vi "sub_lidar-range_line.vi"() -> (3 "guide line":cluster{cluster{"x":dbl, "y":dbl}[]})   [LabVIEW 2019]
uses:
  Ctrl/obstacle_info.ctl
panel:
  in  "input cluster":cluster{"h-L":i16, "h-R":i16}
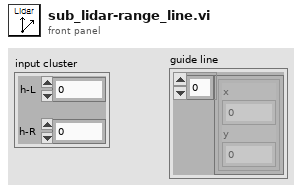
[diagram p1: front panel]
types:
  T1 = typedef "obstacle_info.ctl" = enum16{"init", "read", "obstacle status in", "write limit", "inrange pt-n"}
  T2 = cluster{"h range":cluster{i16, i16}, "v range":cluster{i8, i8}}
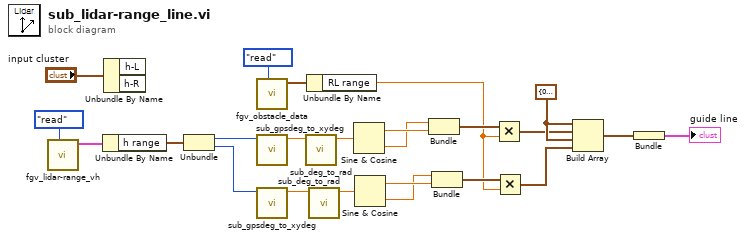
[diagram p0: block diagram]
diagram:
  w22 = cluster{"x":dbl, "y":dbl} {"x"=0.0, "y"=0.0} ("output cluster")
  n1 = call "fgv_lidar-range_vh.vi"("cmd"=enum16{"read", "write"}."read") -> ("VLP16 cfg out"=w4:T2)  [unwired: 10 in]
  n2 = Unbundle By Name(w4) -> ("h range"=w3:cluster{i16, i16})
  n3 = Unbundle By Name("input cluster") -> ()  [unwired: 2 out]
  n4 = Unbundle(w3) -> (w2:i16, w1:i16)
  n5 = call "fgv_obstacle_data.vi"("cmd"=obstacle_info."read") -> ("limit out"=w15:cluster{"RL range":dbl, "Point limit":u16})  [unwired: 7 in, 3 out]
  n6 = call "sub_gpsdeg_to_xydeg.vi"("Heading"=w2) -> ("deg"=w24:dbl)  [unwired: 10 in]
  n7 = call "sub_gpsdeg_to_xydeg.vi"("Heading"=w1) -> ("deg"=w18:dbl)  [unwired: 10 in]
  n8 = call "sub_deg_to_rad.vi"("deg in"=w24) -> ("rad out"=w13:dbl)  [unwired: 10 in]
  n9 = Unbundle By Name(w15) -> ("RL range"=w14:dbl)
  n10 = call "sub_deg_to_rad.vi"("deg in"=w18) -> ("rad out"=w12:dbl)  [unwired: 10 in]
  n11 = Sine & Cosine(0:w13) -> (1:w11:dbl, 2:w10:dbl)
  n12 = Sine & Cosine(0:w12) -> (1:w9:dbl, 2:w8:dbl)
  n13 = Bundle(w10, w11) -> (w23:cluster{dbl, dbl})  [unwired: 1 in]
  n14 = Bundle(w8, w9) -> (w19:cluster{dbl, dbl})  [unwired: 1 in]
  n15 = Multiply(x=w23, y=w14) -> (x*y=w21:cluster{dbl, dbl})
  n16 = Multiply(x=w19, y=w14) -> (x*y=w17:cluster{dbl, dbl})
  n17 = Build Array(w22, w21, w22, w17) -> (w7:cluster{"x":dbl, "y":dbl}[])
  n18 = Bundle(w7) -> (→"guide line":cluster{cluster{"x":dbl, "y":dbl}[]})  [unwired: 1 in]
